vi "State Machine_Pipelined Burst FFT.vi"(5 "FFT Size":T1=enum."8192", 7 "Required FFT Length":u16, 8 "Start FFT (New Record)":bool) -> (0 "Get New Data":bool, 1 "Current Index":u16, 3 "State Info":T3, 4 "FFT SM Current State":T2)   [LabVIEW 2012]
uses:
  <userlib>/FPGA Library/Code Development/Signal Processing/FFT Block/FFT/Controls/FFT States.ctl
  <userlib>/FPGA Library/Code Development/Signal Processing/FFT Block/FFT/FFT Size.ctl
panel:
  out "fwd_inv":bool
  out "fwd_inv_we":bool
  out "Start FFT":bool
  out "Reset":bool
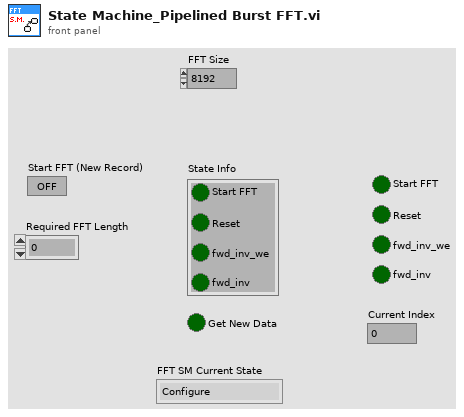
[diagram p1: front panel]
types:
  T1 = typedef "FFT Size.ctl" = enum16{"32", "64", "128", "256", "512", "1024", "2048", "4096", "8192", "16384", "32768", "65536"}
  T2 = typedef "FFT States.ctl" = enum8{"Configure", "Start FFT processing", "Process", "Unload Last FFT", "Reset"}
  T3 = cluster{"Reset":bool, "Start FFT":bool, "fwd_inv_we":bool, "fwd_inv":bool}
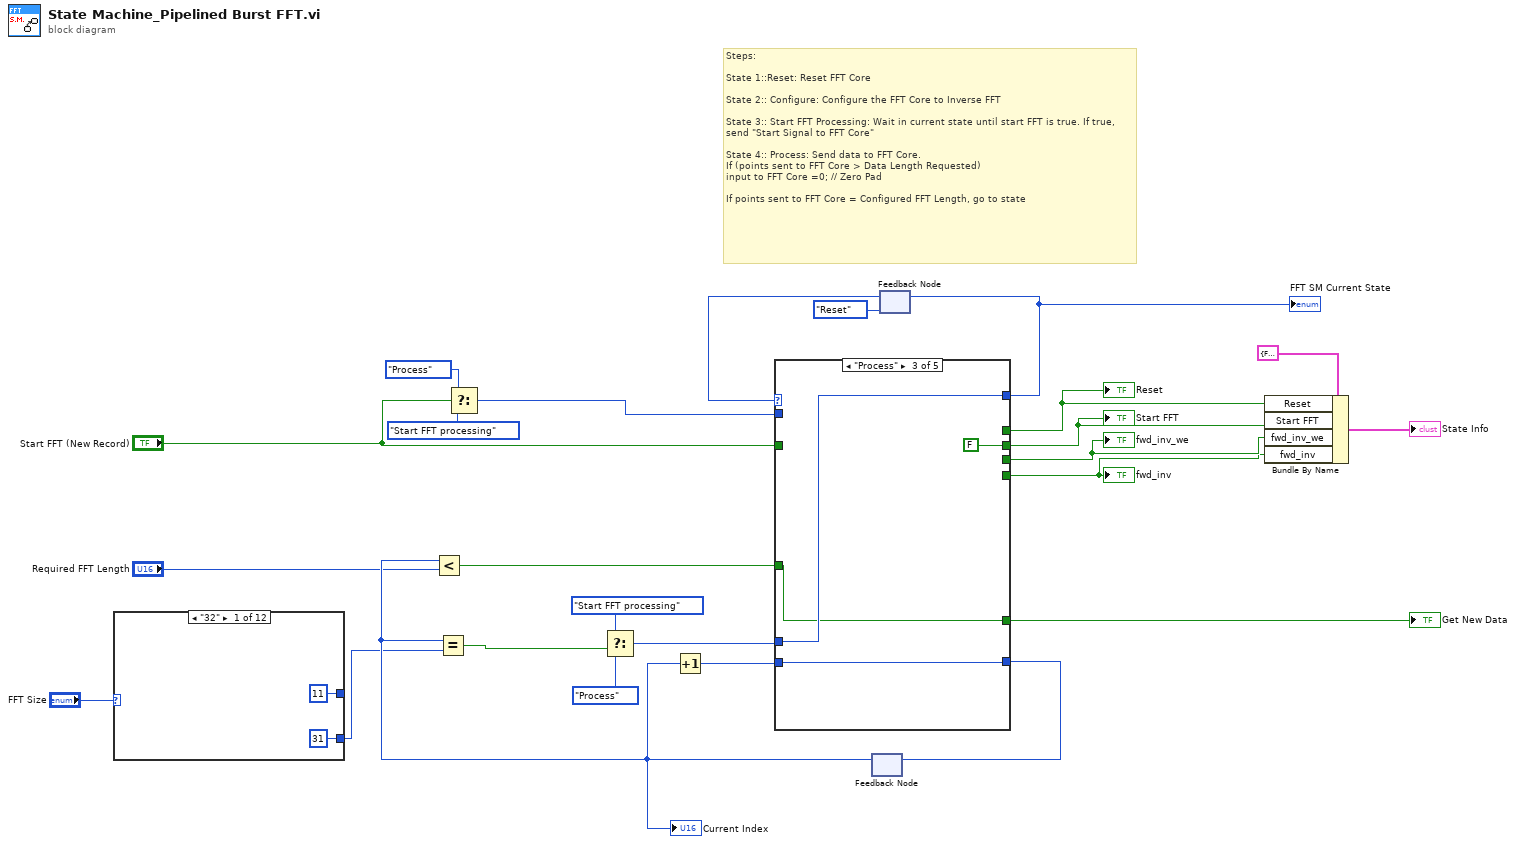
[diagram p0: block diagram]
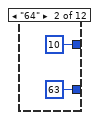
[diagram p2: hidden frame]
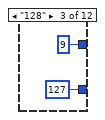
[diagram p3: hidden frame]
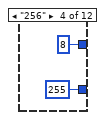
[diagram p4: hidden frame]
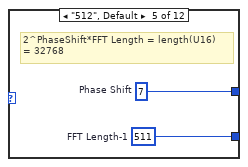
[diagram p5: hidden frame]
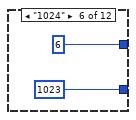
[diagram p6: hidden frame]
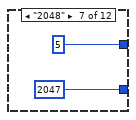
[diagram p7: hidden frame]
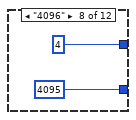
[diagram p8: hidden frame]
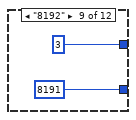
[diagram p9: hidden frame]
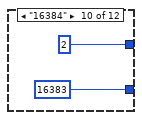
[diagram p10: hidden frame]
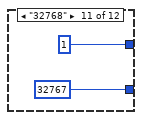
[diagram p11: hidden frame]
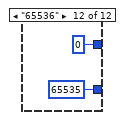
[diagram p12: hidden frame]
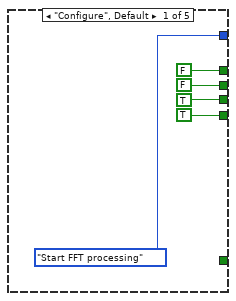
[diagram p13: hidden frame]
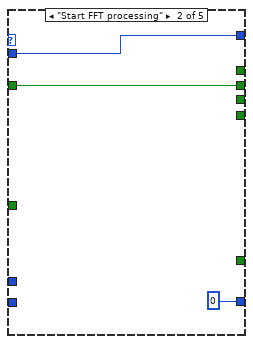
[diagram p14: hidden frame]
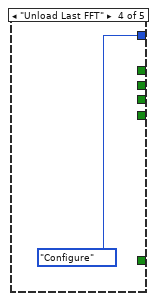
[diagram p15: hidden frame]
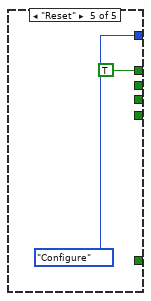
[diagram p16: hidden frame]
diagram:
  # "Steps:\n\nState 1::Reset: Reset FFT Core\n\nState 2:: Configure: Configure the FFT Core to Inverse FFT\n\nState 3:: Start FFT Processing: Wait in current state until start FFT is true. If true, send \"Start Signal to FFT Core\"\n\nState 4:: Process: Send data to FFT Core. \nIf (points sent to FFT Core > Data Length Requested)\ninput to FFT Core =0; // Zero Pad\n\nIf points sent to FFT Core = Configured FFT Length, go to state"
  n1 = case shown="\"32\"" "FFT Size" {
    tunnel: [u8 11 ("n") u8 10 ("n") u8 9 ("n") u8 8 ("n") w35 u8 6 ("n") u8 5 ("n") u8 4 ("n") u8 3 ("n") u8 2 ("n") u8 1 ("n") u8 0 ("n")] -> _
    tunnel: [u16 31 ("FFT Length-1") u16 63 ("FFT Length-1") u16 127 ("FFT Length-1") u16 255 ("FFT Length-1") w34 u16 1023 u16 2047 u16 4095 u16 8191 u16 16383 u16 32767 u16 65535 ("FFT Length-1")] -> w1
    frame "32" {
    }
    frame "64" {
    }
    frame "128" {
    }
    frame "256" {
    }
    frame "512", Default {
      w34 = u16 511  # FFT Length-1
      w35 = u8 7  # Phase Shift
      # "2^PhaseShift*FFT Length = length(U16)\n= 32768"
    }
    frame "1024" {
    }
    frame "2048" {
    }
    frame "4096" {
    }
    frame "8192" {
    }
    frame "16384" {
    }
    frame "32768" {
    }
    frame "65536" {
    }
  }
  n2 = Select(t=FFT_States."Process" ("FFT State"), s="Start FFT (New Record)", f=FFT_States."Start FFT processing") -> (s? t:f=w20:T2)
  n3 = feedback #1() -> (w14:u16)  [unwired: 1 in]
  "Current Index" <- w14
  n4 = Less?(x=w14, y="Required FFT Length") -> (x < y?=w3:bool)
  n5 = Equal?(x=w14, y=w1) -> (x = y?=w6:bool)
  n6 = Select(t=FFT_States."Start FFT processing" ("FFT State"), s=w6, f=FFT_States."Process") -> (s? t:f=w17:T2)
  n7 = Increment(x=w14) -> (x+1=w16:u16)
  n8 = feedback #2(FFT_States."Reset" ("FFT State")) -> (w24:T2)
  n9 = case shown="\"Process\"" w24 {
    tunnel: [FALSE _ _ _ TRUE] -> w12
    tunnel: [FALSE w55 FALSE _ _] -> w11
    tunnel: [FFT_States."Start FFT processing" ("FFT State") w57 w60 FFT_States."Configure" ("f") FFT_States."Configure" ("f")] -> w23
    tunnel: "Start FFT (New Record)" -> [_ w55 _ _ _]
    tunnel: w20 -> [_ w57 _ _ _]
    tunnel: w17 -> [_ _ w60 _ _]
    tunnel: [TRUE ("fwd_inv_we") _ _ _ _] -> w10
    tunnel: [TRUE ("fwd_inv") _ _ _ _] -> w9
    tunnel: w16 -> [_ _ w59 _ _]
    tunnel: [_ u16 0 w59 _ _] -> w15
    tunnel: [_ _ w58 _ _] -> w7
    tunnel: w3 -> [_ _ w58 _ _]
    frame "Configure", Default {
    }
    frame "Start FFT processing" {
    }
    frame "Process" {
    }
    frame "Unload Last FFT" {
    }
    frame "Reset" {
    }
  }
  "Reset" <- w12
  "Start FFT" <- w11
  "fwd_inv_we" <- w10
  "fwd_inv" <- w9
  "FFT SM Current State" <- w23
  "Get New Data" <- w7
  n10 = feedback-in #1(w15) -> ()
  n11 = feedback-in #2(w23) -> ()
  n12 = Bundle By Name(cluster=T3 {"Reset"=FALSE, "Start FFT"=FALSE, "fwd_inv_we"=FALSE, "fwd_inv"=FALSE} ("State Info"), "Reset"=w12, "Start FFT"=w11, "fwd_inv_we"=w10, "fwd_inv"=w9) -> (→"State Info":T3)
